vi "XML Read.vi"(8 "error in":errorcluster, 11 "XML File Path In":path) -> (0 "error out":errorcluster, 3 "FOFB Parameters":T1)   [LabVIEW 2011, in "XML VIs.lvlib"]
doc: "Reads an XML file coitaning the FOFB configuration parameters and builds a raw configuration cluster (FOFB Parameters)."
uses:
  XML VIs.lvlib
  Types Definitions/Type FOFB Parameters.ctl
  Types Definitions/Type Network Configuration.ctl
  Types Definitions/Type FA Configuration.ctl
  Types Definitions/Type Response Matrix Measurement Configuration.ctl
  Types Definitions/Type Correction Algorithm Configuration.ctl
  Types Definitions/Type Acquisition Network Configuration.ctl
  Types Definitions/Type Actuation Network Configuration.ctl
  Third Party/GXML/_subVIis/GXML SearchParser/gxml_SearchParser.vi
  Third Party/GXML/GXML.lvlib
  Type Definitions.lvlib
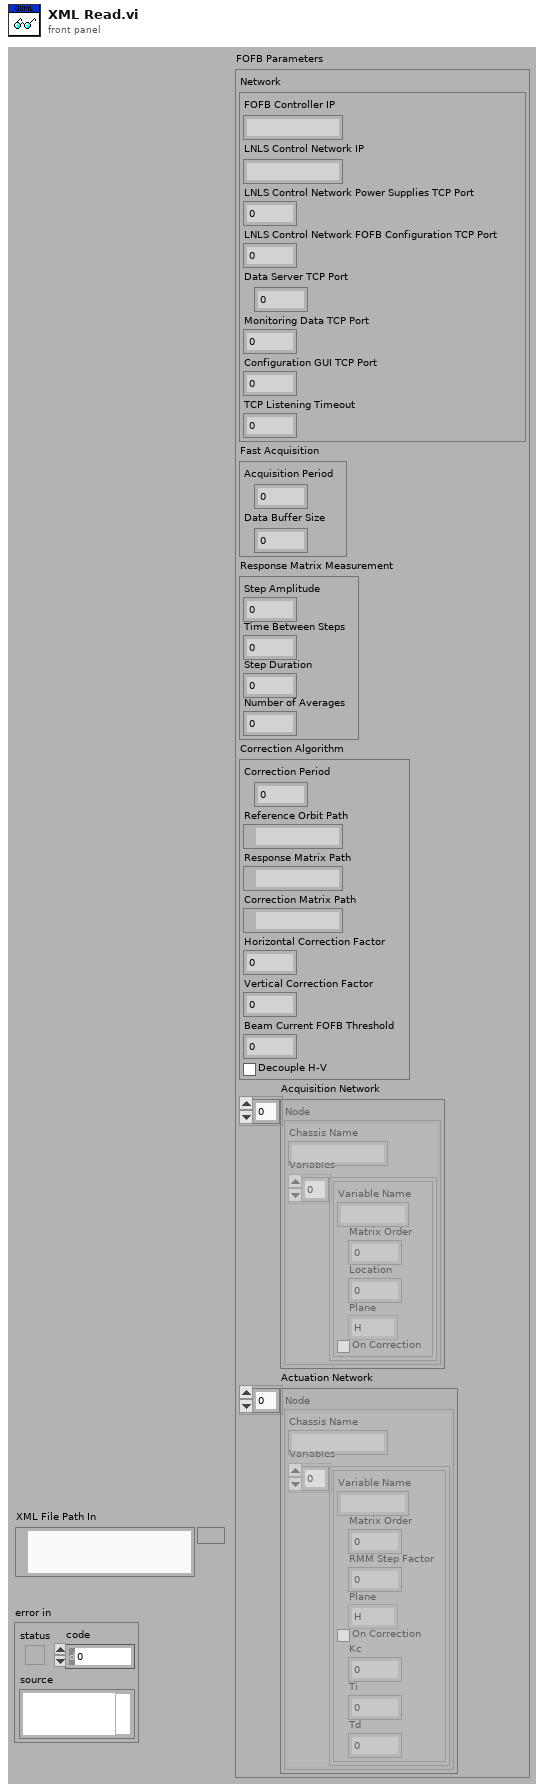
[diagram p1: front panel]
types:
  T1 = typedef "Type Definitions.lvlib/Type FOFB Parameters.ctl" = cluster{"Network":T2, "Fast Acquisition":T3, "Response Matrix Measurement":T4, "Correction Algorithm":T5, "Acquisition Network":T6, "Actuation Network":T7}
  T2 = typedef "Type Definitions.lvlib/Type Network Configuration.ctl" = cluster{"FOFB Controller IP":string, "LNLS Control Network IP":string, "LNLS Control Network Power Supplies TCP Port":u16, "LNLS Control Network FOFB Configuration TCP Port":u16, "Data Server TCP Port":u16, "Monitoring Data TCP Port":u16, "Configuration GUI TCP Port":u16, "TCP Listening Timeout":i32}
  T3 = typedef "Type Definitions.lvlib/Type FA Configuration.ctl" = cluster{"Acquisition Period":u32, "Data Buffer Size":u32}
  T4 = typedef "Type Definitions.lvlib/Type Response Matrix Measurement Configuration.ctl" = cluster{"Step Amplitude":dbl, "Time Between Steps":u32, "Step Duration":u32, "Number of Averages":u32}
  T5 = typedef "Type Definitions.lvlib/Type Correction Algorithm Configuration.ctl" = cluster{"Correction Period":u32, "Reference Orbit Path":path, "Response Matrix Path":path, "Correction Matrix Path":path, "Horizontal Correction Factor":dbl, "Vertical Correction Factor":dbl, "Beam Current FOFB Threshold":dbl, "Decouple H-V":bool}
  T6 = typedef "Type Definitions.lvlib/Type Acquisition Network Configuration.ctl" = cluster{"Chassis Name":string, "Variables":cluster{"Variable Name":string, "Matrix Order":u32, "Location":dbl, "Plane":enum8{"H", "V"}, "On Correction":bool}[]}[]
  T7 = typedef "Type Definitions.lvlib/Type Actuation Network Configuration.ctl" = cluster{"Chassis Name":string, "Variables":cluster{"Variable Name":string, "Matrix Order":u32, "RMM Step Factor":dbl, "Plane":enum8{"H", "V"}, "On Correction":bool, "Kc":dbl, "Ti":dbl, "Td":dbl}[]}[]
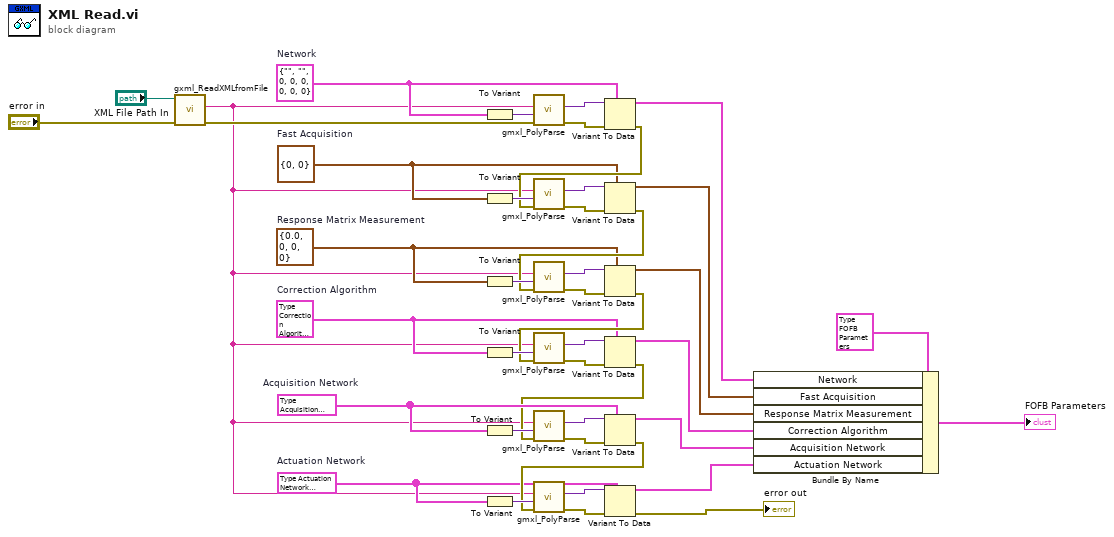
[diagram p0: block diagram]
diagram:
  w2 = T5 {"Correction Period"=0, "Reference Orbit Path"=path "", "Response Matrix Path"=path "", "Correction Matrix Path"=path "", "Horizontal Correction Factor"=0.0, "Vertical Correction Factor"=0.0, "Beam Current FOFB Threshold"=0.0, "Decouple H-V"=FALSE}  # Correction Algorithm
  w8 = T3 {"Acquisition Period"=0, "Data Buffer Size"=0}  # Fast Acquisition
  w9 = T2 {"FOFB Controller IP"="", "LNLS Control Network IP"="", "LNLS Control Network Power Supplies TCP Port"=0, "LNLS Control Network FOFB Configuration TCP Port"=0, "Data Server TCP Port"=0, "Monitoring Data TCP Port"=0, "Configuration GUI TCP Port"=0, "TCP Listening Timeout"=0}  # Network
  w5 = T4 {"Step Amplitude"=0.0, "Time Between Steps"=0, "Step Duration"=0, "Number of Averages"=0}  # Response Matrix Measurement
  w32 = T7 [{"Chassis Name"="", "Variables"=[{"Variable Name"="", "Matrix Order"=0, "RMM Step Factor"=0.0, "Plane"=enum."H", "On Correction"=FALSE, "Kc"=0.0, "Ti"=0.0, "Td"=0.0}, {"Variable Name"="", "Matrix Order"=0, "RMM Step Factor"=0.0, "Plane"=enum."H", "On Correction"=FALSE, "Kc"=0.0, "Ti"=0.0, "Td"=0.0}, {"Variable Name"="", "Matrix Order"=0, "RMM Step Factor"=0.0, "Plane"=enum."H", "On Correction"=FALSE, "Kc"=0.0, "Ti"=0.0, "Td"=0.0}, {"Variable Name"="", "Matrix Order"=0, "RMM Step Factor"=0.0, "Plane"=enum."H", "On Correction"=FALSE, "Kc"=0.0, "Ti"=0.0, "Td"=0.0}, {"Variable Name"="", "Matrix Order"=0, "RMM Step Factor"=0.0, "Plane"=enum."H", "On Correction"=FALSE, "Kc"=0.0, "Ti"=0.0, "Td"=0.0}, {"Variable Name"="", "Matrix Order"=0, "RMM Step Factor"=0.0, "Plane"=enum."H", "On Correction"=FALSE, "Kc"=0.0, "Ti"=0.0, "Td"=0.0}, {"Variable Name"="", "Matrix Order"=0, "RMM Step Factor"=0.0, "Plane"=enum."H", "On Correction"=FALSE, "Kc"=0.0, "Ti"=0.0, "Td"=0.0}, {"Variable Name"="", "Matrix Order"=0, "RMM Step Factor"=0.0, "Plane"=enum."H", "On Correction"=FALSE, "Kc"=0.0, "Ti"=0.0, "Td"=0.0}]}]  # Actuation Network
  w33 = T6 [{"Chassis Name"="", "Variables"=[{"Variable Name"="", "Matrix Order"=0, "Location"=0.0, "Plane"=enum."H", "On Correction"=FALSE}, {"Variable Name"="", "Matrix Order"=0, "Location"=0.0, "Plane"=enum."H", "On Correction"=FALSE}, {"Variable Name"="", "Matrix Order"=0, "Location"=0.0, "Plane"=enum."H", "On Correction"=FALSE}, {"Variable Name"="", "Matrix Order"=0, "Location"=0.0, "Plane"=enum."H", "On Correction"=FALSE}, {"Variable Name"="", "Matrix Order"=0, "Location"=0.0, "Plane"=enum."H", "On Correction"=FALSE}, {"Variable Name"="", "Matrix Order"=0, "Location"=0.0, "Plane"=enum."H", "On Correction"=FALSE}, {"Variable Name"="", "Matrix Order"=0, "Location"=0.0, "Plane"=enum."H", "On Correction"=FALSE}, {"Variable Name"="", "Matrix Order"=0, "Location"=0.0, "Plane"=enum."H", "On Correction"=FALSE}]}]  # Acquisition Network
  n1 = call "gxml_ReadXMLfromFile.vi"("error in"="error in", "XML File Path"="XML File Path In") -> ("error out"=w17:errorcluster, "XML String Out"=w1:string)  [unwired: 7 in, 1 out]
  n2 = To Variant(anything=w9) -> (Variant=w18:variant)
  n3 = To Variant(anything=w8) -> (Variant=w23:variant)
  n4 = To Variant(anything=w5) -> (Variant=w29:variant)
  n5 = To Variant(anything=w2) -> (Variant=w28:variant)
  n6 = To Variant(anything=w33) -> (Variant=w41:variant)
  n7 = To Variant(anything=w32) -> (Variant=w36:variant)
  n8 = call-poly "gmxl_PolyParse.vi"("error in"=w17, "TypeDesc"=w18, "XML String In"=w1) -> ("error out"=w20:errorcluster, "Parsed Data"=w19:variant)  [unwired: 7 in]
  n9 = Variant To Data(error in=w20, type=w9, Variant=w19) -> (data=w6:T2, error out=w16:errorcluster)
  n10 = call-poly "gmxl_PolyParse.vi"("error in"=w16, "TypeDesc"=w23, "XML String In"=w1) -> ("error out"=w21:errorcluster, "Parsed Data"=w22:variant)  [unwired: 7 in]
  n11 = Variant To Data(error in=w21, type=w8, Variant=w22) -> (data=w7:T3, error out=w10:errorcluster)
  n12 = call-poly "gmxl_PolyParse.vi"("error in"=w10, "TypeDesc"=w29, "XML String In"=w1) -> ("error out"=w31:errorcluster, "Parsed Data"=w30:variant)  [unwired: 7 in]
  n13 = Variant To Data(error in=w31, type=w5, Variant=w30) -> (data=w3:T4, error out=w25:errorcluster)
  n14 = call-poly "gmxl_PolyParse.vi"("error in"=w25, "TypeDesc"=w28, "XML String In"=w1) -> ("error out"=w26:errorcluster, "Parsed Data"=w27:variant)  [unwired: 7 in]
  n15 = Variant To Data(error in=w26, type=w2, Variant=w27) -> (data=w4:T5, error out=w24:errorcluster)
  n16 = call-poly "gmxl_PolyParse.vi"("error in"=w24, "TypeDesc"=w41, "XML String In"=w1) -> ("error out"=w39:errorcluster, "Parsed Data"=w40:variant)  [unwired: 7 in]
  n17 = Variant To Data(error in=w39, type=w33, Variant=w40) -> (data=w13:T6, error out=w35:errorcluster)
  n18 = call-poly "gmxl_PolyParse.vi"("error in"=w35, "TypeDesc"=w36, "XML String In"=w1) -> ("error out"=w38:errorcluster, "Parsed Data"=w37:variant)  [unwired: 7 in]
  n19 = Variant To Data(error in=w38, type=w32, Variant=w37) -> (data=w14:T7, error out=→"error out":errorcluster)
  n20 = Bundle By Name(cluster=T1 {"Network"={"FOFB Controller IP"="", "LNLS Control Network IP"="", "LNLS Control Network Power Supplies TCP Port"=0, "LNLS Control Network FOFB Configuration TCP Port"=0, "Data Server TCP Port"=0, "Monitoring Data TCP Port"=0, "Configuration GUI TCP Port"=0, "TCP Listening Timeout"=0}, "Fast Acquisition"={"Acquisition Period"=0, "Data Buffer Size"=0}, "Response Matrix Measurement"={"Step Amplitude"=0.0, "Time Between Steps"=0, "Step Duration"=0, "Number of Averages"=0}, "Correction Algorithm"={"Correction Period"=0, "Reference Orbit Path"=path "", "Response Matrix Path"=path "", "Correction Matrix Path"=path "", "Horizontal Correction Factor"=0.0, "Vertical Correction Factor"=0.0, "Beam Current FOFB Threshold"=0.0, "Decouple H-V"=FALSE}, "Acquisition Network"=[], "Actuation Network"=[]} ("FOFB Parameters"), "Network"=w6, "Fast Acquisition"=w7, "Response Matrix Measurement"=w3, "Correction Algorithm"=w4, "Acquisition Network"=w13, "Actuation Network"=w14) -> (→"FOFB Parameters":T1)
